vi "FRead.vi"(5 "error in (no error)":errorcluster, 6 "File ID":string, 7 "仪器地址":u32, 8 "VISA resource name in":refnum<visa-resource-name>) -> (0 "error out":errorcluster, 1 "Segment 0":T2, 2 "Segment 1 to 99":T1(array[cluster]), 3 "VISA resource name out":refnum<visa-resource-name>)   [LabVIEW 2010, in "DCP551.lvlib"]
uses:
  DCP551.lvlib
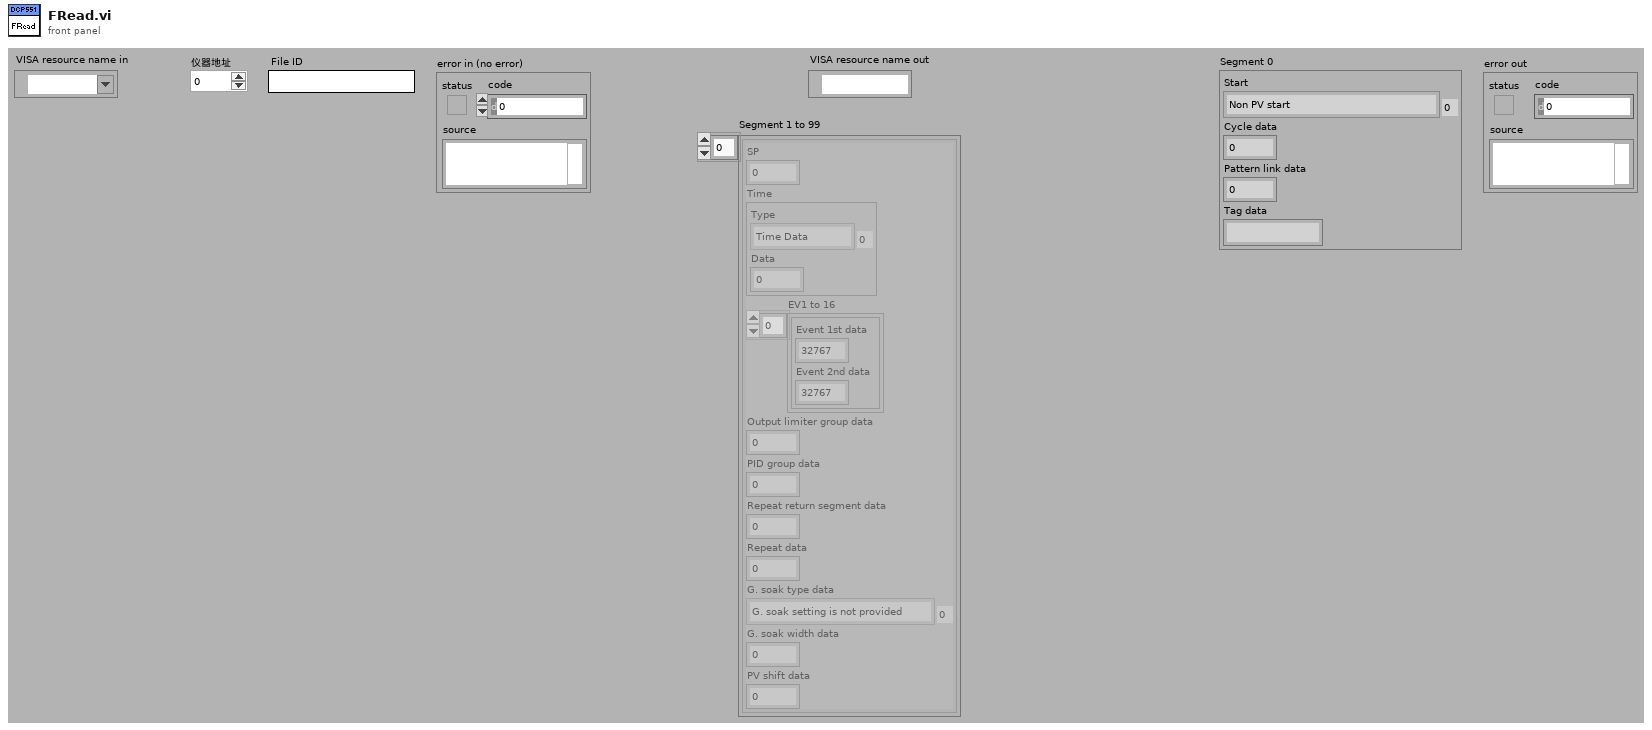
[diagram p1: front panel]
types:
  T1 = cluster{"SP":dbl, "Time":cluster{"Type":enum16{"Time Data", "delta Dtada", "SP Data"}, "Data":i32}, "EV1 to 16":cluster{"Event 1st data":i32, "Event 2nd data":i32}[], "Output limiter group data":i32, "PID group data":i32, "Repeat return segment data":i32, "Repeat data":i32, "G. soak type data":enum16{"G. soak setting is not provided", "Segment start point", "Segment end point", "Total segment"}, "G. soak width data":i32, "PV shift data":i32}[]
  T2 = cluster{"Start":enum16{"Non PV start", "Upward PV tart", "Downward PV start", "Either upward of downward PV start"}, "Cycle data":i32, "Pattern link data":i32, "Tag data":string}
  T3 = cluster{"SP":dbl, "Time":cluster{"Type":enum16{"Time Data", "delta Dtada", "SP Data"}, "Data":i32}, "EV1 to 16":cluster{"Event 1st data":i32, "Event 2nd data":i32}[], "Output limiter group data":i32, "PID group data":i32, "Repeat return segment data":i32, "Repeat data":i32, "G. soak type data":enum16{"G. soak setting is not provided", "Segment start point", "Segment end point", "Total segment"}, "G. soak width data":i32, "PV shift data":i32}
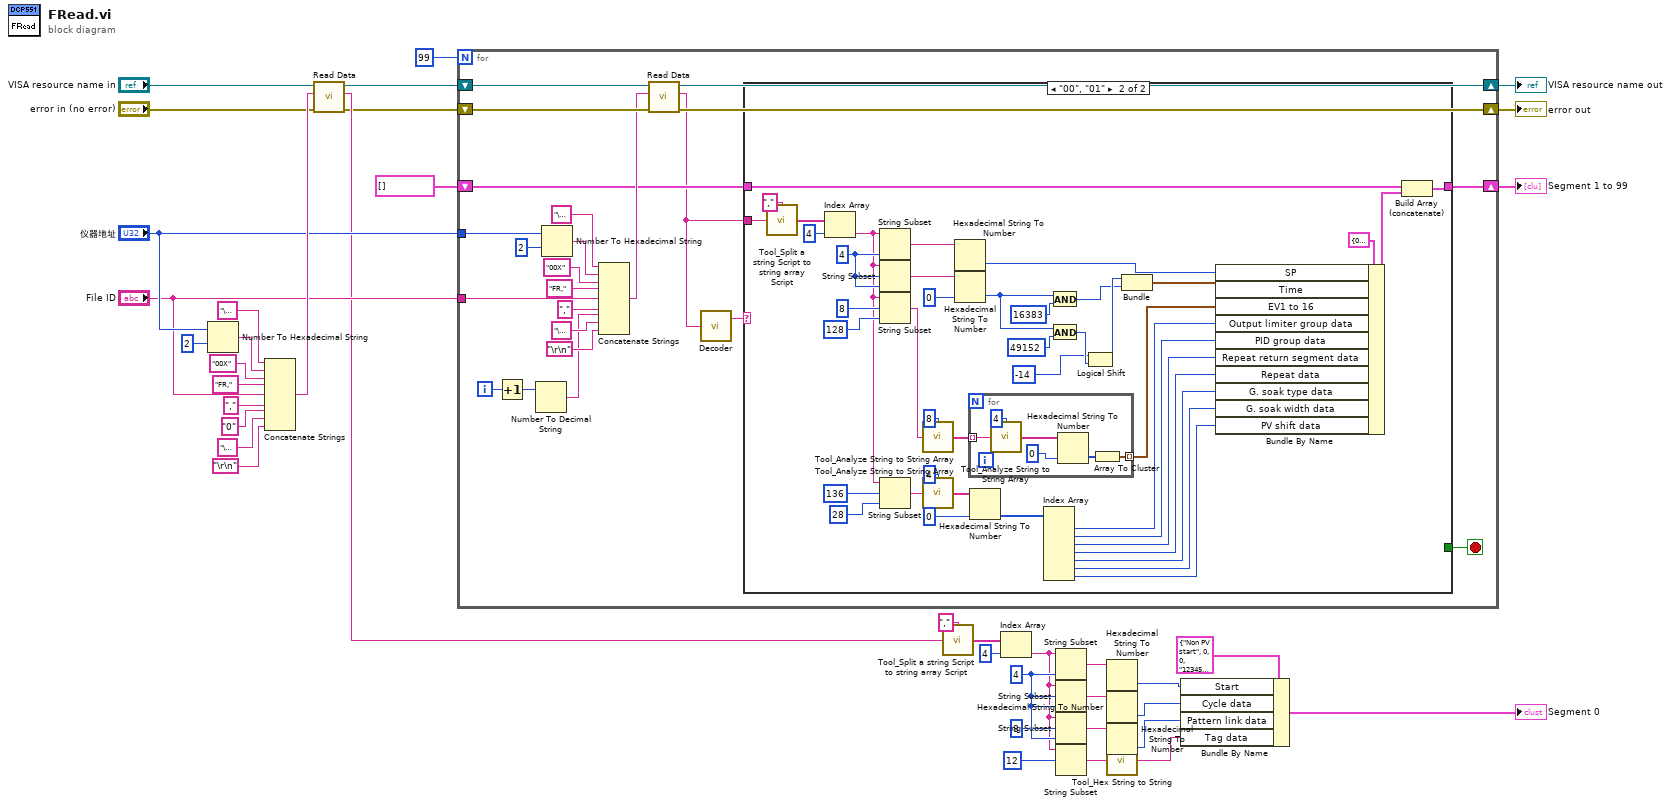
[diagram p0: block diagram]
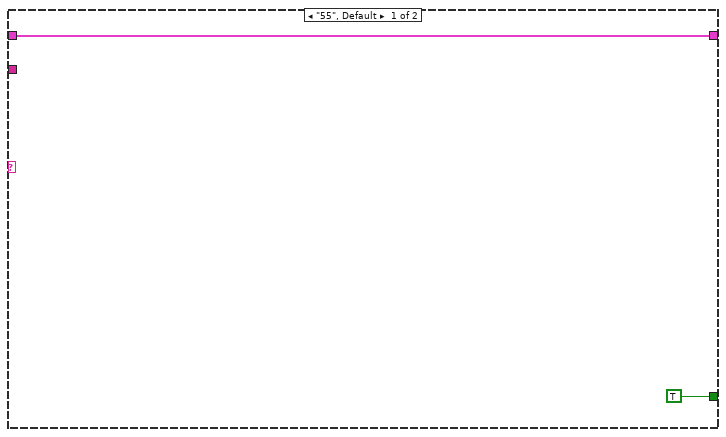
[diagram p2: hidden frame]
diagram:
  w12 = 4 ("length (rest)")
  n1 = Number To Hexadecimal String(1:i16 2 ("width (-)"), 2:"仪器地址") -> (0:w34:string)
  n2 = Concatenate Strings("\u0002" ("string"), w34, "00X" ("string"), "FR," ("string"), "File ID", "," ("string"), "0" ("string"), "\u0003" ("string"), "\r\n") -> (w28:string)
  n3 = call "Read Data.vi"("error in (no error)"="error in (no error)", "COMMAND"=w28, "VISA resource name in"="VISA resource name in") -> ("error out"=w5:errorcluster, "Output"=w6:string, "VISA resource name out"=w4:refnum<visa-resource-name>)  [unwired: 6 in]
  n4 = for {
    N: 99 -> [_]
    tunnel: "File ID" -> [w60]
    tunnel: "仪器地址" -> [w59]
    shift-right: [w61] -> w38
    shift-left: w4 -> [w56]
    shift-right: [w62] -> w39
    shift-left: w5 -> [w58]
    shift-right: [w43] -> w2
    shift-left: T1 [] -> [w42]
    i -> [w46]
    stop <- w41 stop-if-true
    n5 = Increment(x=w46) -> (x+1=w45:i32)
    n6 = Number To Decimal String(number=w45) -> (decimal integer string=w47:string)  [unwired: 1 in]
    n7 = Number To Hexadecimal String(1:i16 2 ("width (-)"), 2:w59) -> (0:w50:string)
    n8 = Concatenate Strings("\u0002" ("string"), w50, "00X" ("string"), "FR," ("string"), w60, "," ("string"), w47, "\u0003" ("string"), "\r\n") -> (w57:string)
    n9 = call "Read Data.vi"("error in (no error)"=w58, "COMMAND"=w57, "VISA resource name in"=w56) -> ("error out"=w62:errorcluster, "Output"=w40:string, "VISA resource name out"=w61:refnum<visa-resource-name>)  [unwired: 6 in]
    n10 = call "Decoder.vi"("Input"=w40) -> ("Status Code"=w44:string)  [unwired: 1 out]
    n11 = case shown="\"00\", \"01\"" w44 {
      tunnel: w40 -> [_ w106]
      tunnel: [w64 w67] -> w43
      tunnel: w42 -> [w64 w66]
      tunnel: [TRUE _] -> w41
      frame "55", Default {
      }
      frame "00", "01" {
        w101 = 4 ("length (rest)")
        n12 = call "Tool_Split a string Script to string array Script.vi"("search string"=",", "input string"=w106) -> ("Array"=w104:string[])  [unwired: 13 in]
        n13 = Index Array(array=w104, index=4) -> (element=w82:string)
        n14 = String Subset(string=w82, length (rest)=w101) -> (substring=w93:string)  [unwired: 1 in]
        n15 = String Subset(string=w82, offset (0)=w101, length (rest)=w101) -> (substring=w91:string)
        n16 = String Subset(string=w82, offset (0)=8, length (rest)=128 ("length (rest)")) -> (substring=w87:string)
        n17 = String Subset(string=w82, offset (0)=136, length (rest)=28 ("length (rest)")) -> (substring=w79:string)
        n18 = call "Tool_Analyze String to String Array.vi"("Length (1)"=8, "String"=w87) -> ("String Array"=w85:string[])  [unwired: 13 in]
        n19 = call "Tool_Analyze String to String Array.vi"("Length (1)"=4, "String"=w79) -> ("String Array"=w78:string[])  [unwired: 13 in]
        n20 = Hexadecimal String To Number(string=w93) -> (number=w92:u32)  [unwired: 2 in, 1 out]
        n21 = Hexadecimal String To Number(string=w91, default (0uL)=u16 0 ("Cycle data")) -> (number=w89:u16)  [unwired: 1 in, 1 out]
        n22 = for {
          tunnel: w85 -> [w112] mode=indexing
          tunnel: [w107] -> w84 mode=indexing
          n23 = call "Tool_Analyze String to String Array.vi"("Length (1)"=4, "String"=w112) -> ("String Array"=w109:string[])  [unwired: 13 in]
          n24 = Hexadecimal String To Number(string=w109, default (0uL)=u16 0 ("Cycle data")) -> (number=w108:u16[])  [unwired: 1 in, 1 out]
          n25 = Array To Cluster(array=w108) -> (cluster=w107:cluster{"[0]":u16, "[1]":u16})
        }
        n26 = Hexadecimal String To Number(string=w78, default (0uL)=u16 0 ("Cycle data")) -> (number=w77:u16[])  [unwired: 1 in, 1 out]
        n27 = Index Array(array=w77) -> (element #1=w76:u16, element #2=w75:u16, element #3=w74:u16, element #4=w73:u16, element #5=w72:u16, element #6=w71:u16, element #7=w70:u16)  [unwired: 7 in]
        n28 = And(x=w89, y=u16 16383) -> (x .and. y?=w95:u16)
        n29 = And(x=w89, y=u16 49152) -> (x .and. y?=w98:u16)
        n30 = Logical Shift(y=i8 -14, x=w98) -> (x << y=w96:u16)
        n31 = Bundle(w96, w95) -> (w94:cluster{u16, u16})  [unwired: 1 in]
        n32 = Bundle By Name(cluster=T3 {"SP"=0.0, "Time"={"Type"=enum."Time Data", "Data"=0}, "EV1 to 16"=[], "Output limiter group data"=0, "PID group data"=0, "Repeat return segment data"=0, "Repeat data"=0, "G. soak type data"=enum."G. soak setting is not provided", "G. soak width data"=0, "PV shift data"=0} ("Segment 1 to 99"), "SP"=w92, "Time"=w94, "EV1 to 16"=w84, "Output limiter group data"=w76, "PID group data"=w75, "Repeat return segment data"=w74, "Repeat data"=w73, "G. soak type data"=w72, "G. soak width data"=w71, "PV shift data"=w70) -> (w68:T3)
        n33 = Build Array (concatenate)(w66, w68) -> (w67:T1)
      }
    }
  }
  "error out" <- w39
  "VISA resource name out" <- w38
  "Segment 1 to 99" <- w2
  n34 = call "Tool_Split a string Script to string array Script.vi"("search string"=",", "input string"=w6) -> ("Array"=w8:string[])  [unwired: 13 in]
  n35 = Index Array(array=w8, index=4) -> (element=w10:string)
  n36 = String Subset(string=w10, length (rest)=w12) -> (substring=w15:string)  [unwired: 1 in]
  n37 = String Subset(string=w10, offset (0)=w12, length (rest)=w12) -> (substring=w17:string)
  n38 = String Subset(string=w10, offset (0)=8, length (rest)=w12) -> (substring=w19:string)
  n39 = String Subset(string=w10, offset (0)=12) -> (substring=w21:string)  [unwired: 1 in]
  n40 = Hexadecimal String To Number(string=w15) -> (number=w16:u32)  [unwired: 2 in, 1 out]
  n41 = Hexadecimal String To Number(string=w17) -> (number=w18:u32)  [unwired: 2 in, 1 out]
  n42 = Hexadecimal String To Number(string=w19) -> (number=w20:u32)  [unwired: 2 in, 1 out]
  n43 = call "Tool_Hex String to String.vi"("Hex String"=w21) -> ("String"=w22:string)  [unwired: 14 in]
  n44 = Bundle By Name(cluster=T2 {"Start"=enum."Non PV start", "Cycle data"=0, "Pattern link data"=0, "Tag data"="12345678"} ("Segment 0"), "Start"=w16, "Cycle data"=w18, "Pattern link data"=w20, "Tag data"=w22) -> (→"Segment 0":T2)
